vi "service_error_parse.vi"(0 "Reply":string="\u0000\u0000\u0000\u0000\u0000") -> (1 "OK?":bool, 2 "Error Code":i32)   [LabVIEW 2012]
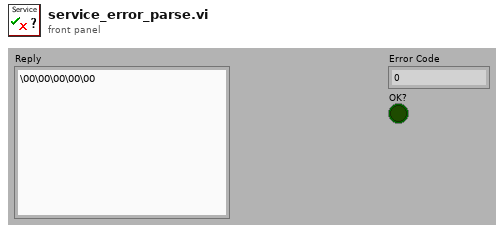
[diagram p1: front panel]
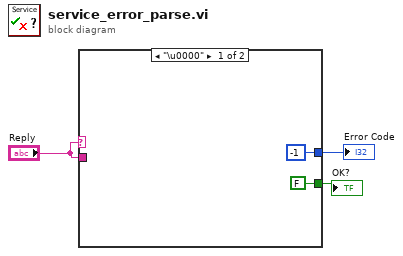
[diagram p0: block diagram]
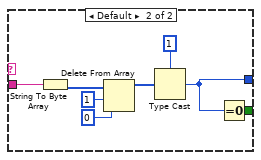
[diagram p2: hidden frame]
diagram:
  n1 = case shown="\"\"" "Reply" {
    tunnel: "Reply" -> [_ w13]
    tunnel: [-1 ("length") w7] -> w3
    tunnel: [FALSE w6] -> w2
    frame "\u0000" {
    }
    frame Default {
      n2 = String To Byte Array(string=w13) -> (unsigned byte array=w12:u8[])
      n3 = Delete From Array(array=w12, length=1, index=0) -> (array with subset deleted=w9:u8[])  [unwired: 1 out]
      n4 = Type Cast(type=1 ("length"), x=w9) -> (*(type *) &x=w7:i32)
      n5 = Equal To 0?(x=w7) -> (x = 0?=w6:bool)
    }
  }
  "Error Code" <- w3
  "OK?" <- w2
